vi "Evaluate Part 1_rev2.vi"() -> ()   [LabVIEW 2020]
uses:
  Range/Range.lvclass
  Map/Map.lvclass
  Range Map/Range Map.lvclass
panel:
  out "min value":u32
  in  "Input":string="seeds: 79 14 55 13\n\nseed-to-soil map:\n50 98 2\n52 50 48\n\nsoil-to-fertilizer map:\n0 15 37\n37 52 2\n39 0 15\n\nfertilizer-to-water map:\n49 53 8\n0 11 42\n42 0 7\n57 7 4\n\nwater-to-light map:\n88 18 7\n18 25 70\n\nlight-to-temperature map:\n45 77 23\n81 45 19\n68 64 13\n\ntemperature-to-humidity map:\n0 69 1\n1 0 69\n\nhumidity-to-location map:\n60 56 37\n56 93 4"
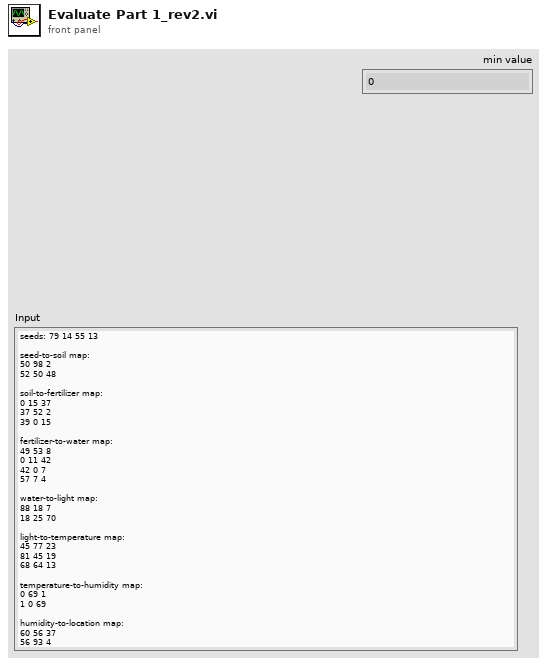
[diagram p1: front panel]
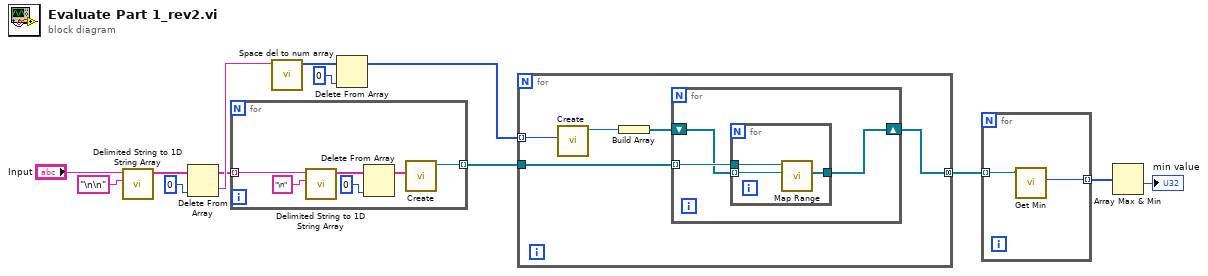
[diagram p0: block diagram]
diagram:
  n1 = call <vilib>:"Delimited String to 1D String Array.vi"("delimiter"="\n\n" ("String"), "delimited string"="Input") -> ("string array"=w7:string[])  [unwired: 9 in]
  n2 = Delete From Array(array=w7, index=0) -> (deleted portion=w10:string, array with subset deleted=w6:string[])  [unwired: 1 in]
  n3 = for {
    tunnel: w6 -> [w17] mode=indexing
    tunnel: [w14] -> w5 mode=indexing
    n4 = call <vilib>:"Delimited String to 1D String Array.vi"("delimiter"="\n" ("String"), "delimited string"=w17) -> ("string array"=w16:string[])  [unwired: 9 in]
    n5 = Delete From Array(array=w16, index=0) -> (array with subset deleted=w15:string[])  [unwired: 1 in, 1 out]
    n6 = call "Create.vi"("Input"=w15) -> ("Range Map"=w14:refnum<class "Range Map.lvclass">)  [unwired: 9 in, 1 out]
  }
  n7 = call "Space del to num array.vi"("Input in"=w10) -> ("Input out"=w9:u64[])  [unwired: 10 in]
  n8 = Delete From Array(array=w9, index=0) -> (array with subset deleted=w4:u64[])  [unwired: 1 in, 1 out]
  n9 = for {
    tunnel: w5 -> [w24]
    tunnel: w4 -> [w23] mode=indexing
    tunnel: [w20] -> w1 mode=concatenating
    n10 = call "Create.vi"("From"=w23) -> ("Range"=w22:refnum<class "Range.lvclass">)  [unwired: 9 in, 1 out]
    n11 = Build Array(w22) -> (w21:refnum<class "Range.lvclass">[])
    n12 = for {
      tunnel: w24 -> [w27] mode=indexing
      shift-right: [w25] -> w20
      shift-left: w21 -> [w26]
      n13 = for {
        tunnel: w27 -> [w30]
        tunnel: w26 -> [w29] mode=indexing
        tunnel: [w28] -> w25
        n14 = call "Map Range.vi"("Range"=w29, "Range Map in"=w30) -> ("Ranges"=w28:refnum<class "Range.lvclass">[])  [unwired: 7 in, 2 out]
      }
    }
  }
  n15 = for {
    tunnel: [w32] -> w2 mode=indexing
    tunnel: w1 -> [w31] mode=indexing
    n16 = call "Get Min.vi"("Range in"=w31) -> ("Min"=w32:u64)  [unwired: 8 in, 2 out]
  }
  n17 = Array Max & Min(array=w2) -> (min value=→"min value":u64)  [unwired: 3 out]
